vi "client_sw.vi"(5 "receive?":bool, 7 "data in":string, 8 "error constant":errorcluster, 11 "port":u16=6340) -> (0 "error constant 2":errorcluster, 3 "data out":string)   [LabVIEW 2015]
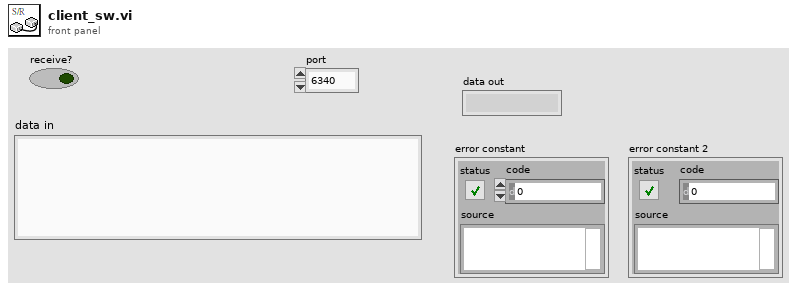
[diagram p1: front panel]
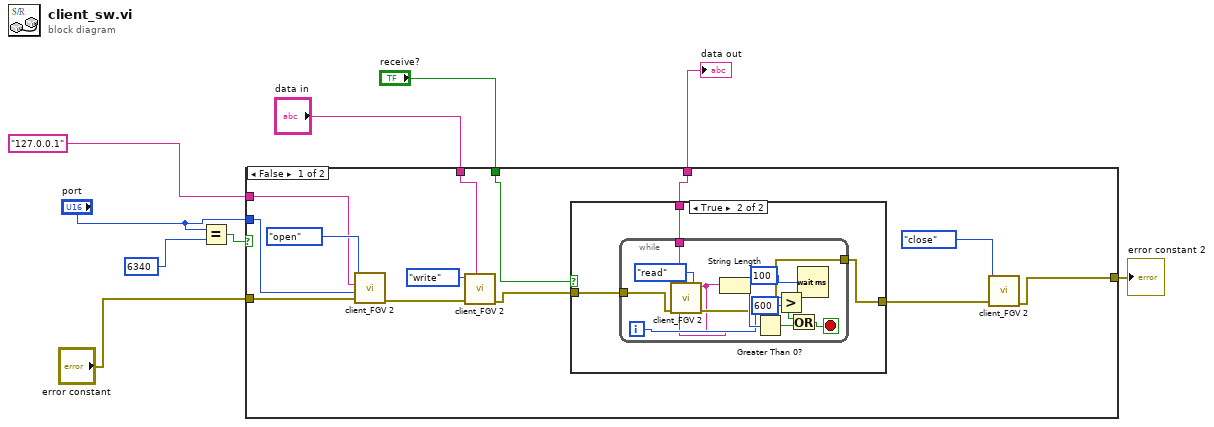
[diagram p0: block diagram]
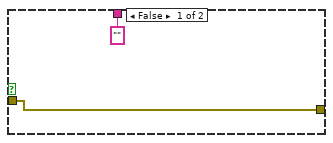
[diagram p2: hidden frame]
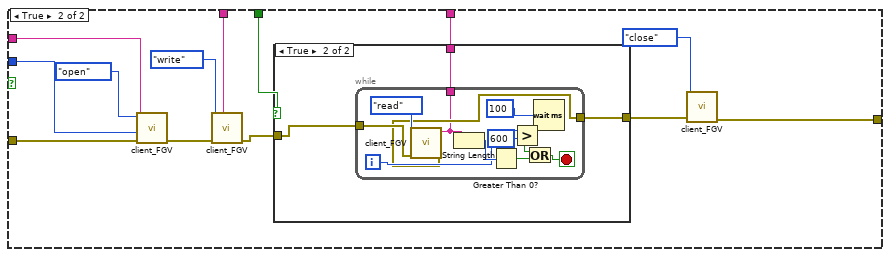
[diagram p3: hidden frame]
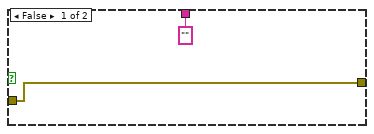
[diagram p4: hidden frame]
diagram:
  n1 = Equal?(x="port", y=u16 6340 ("port")) -> (x = y?=w8:bool)
  n2 = case shown="False" w8 {
    tunnel: "127.0.0.1" ("address") -> [w10 w51]
    tunnel: "port" -> [w11 w50]
    tunnel: "error constant" -> [w20 w49]
    tunnel: "data in" -> [w13 w46]
    tunnel: "receive?" -> [w14 w44]
    tunnel: [w12 w43] -> w2
    tunnel: [w15 w40] -> w1
    frame False {
      n3 = call "client_FGV 2.vi"("error constant"=w20, "port"=w11, "address"=w10, "Enum"=enum16{"open", "idle", "write", "read", "close"}."open") -> ("error constant 2"=w19:errorcluster)  [unwired: 6 in, 1 out]
      n4 = call "client_FGV 2.vi"("data in"=w13, "error constant"=w19, "Enum"=enum16{"open", "idle", "write", "read", "close"}."write") -> ("error constant 2"=w17:errorcluster)  [unwired: 7 in, 1 out]
      n5 = case shown="True" w14 {
        tunnel: w17 -> [w23 w27]
        tunnel: [w23 w26] -> w16
        tunnel: ["" ("data out") w25] -> w12
        frame False {
        }
        frame True {
          n6 = while {
            tunnel: w27 -> [w31]
            tunnel: [w29] -> w26
            tunnel: [w28] -> w25
            i -> [w33]
            stop <- w35 stop-if-true
            n7 = call "client_FGV 2.vi"("error constant"=w31, "Enum"=enum16{"open", "idle", "write", "read", "close"}."read") -> ("error constant 2"=w29:errorcluster, "data out"=w28:string)  [unwired: 8 in]
            n8 = String Length(string=w28) -> (length=w37:i32)
            n9 = Greater Than 0?(x=w37) -> (x > 0?=w36:bool)
            n10 = Greater?(x=w33, y=600) -> (0:w34:bool)
            n11 = Or(x=w34, y=w36) -> (x .or. y?=w35:bool)
            n12 = Wait (ms)(milliseconds to wait=u32 100) -> ()  [unwired: 1 out]
          }
        }
      }
      n13 = call "client_FGV 2.vi"("error constant"=w16, "Enum"=enum16{"open", "idle", "write", "read", "close"}."close") -> ("error constant 2"=w15:errorcluster)  [unwired: 8 in, 1 out]
    }
    frame True {
      n14 = call "client_FGV.vi"("error constant"=w49, "port"=w50, "address"=w51, "Enum"=enum16{"open", "idle", "write", "read", "close"}."open") -> ("error constant 2"=w48:errorcluster)  [unwired: 6 in, 1 out]
      n15 = call "client_FGV.vi"("data in"=w46, "error constant"=w48, "Enum"=enum16{"open", "idle", "write", "read", "close"}."write") -> ("error constant 2"=w45:errorcluster)  [unwired: 7 in, 1 out]
      n16 = case shown="True" w44 {
        tunnel: w45 -> [w53 w56]
        tunnel: ["" ("data out") w55] -> w43
        tunnel: [w53 w54] -> w42
        frame False {
        }
        frame True {
          n17 = while {
            tunnel: w56 -> [w67]
            tunnel: [w58] -> w54
            tunnel: [w57] -> w55
            i -> [w60]
            stop <- w62 stop-if-true
            n18 = call "client_FGV.vi"("error constant"=w67, "Enum"=enum16{"open", "idle", "write", "read", "close"}."read") -> ("error constant 2"=w58:errorcluster, "data out"=w57:string)  [unwired: 8 in]
            n19 = String Length(string=w57) -> (length=w64:i32)
            n20 = Greater Than 0?(x=w64) -> (x > 0?=w63:bool)
            n21 = Greater?(x=w60, y=600) -> (0:w61:bool)
            n22 = Or(x=w61, y=w63) -> (x .or. y?=w62:bool)
            n23 = Wait (ms)(milliseconds to wait=u32 100) -> ()  [unwired: 1 out]
          }
        }
      }
      n24 = call "client_FGV.vi"("error constant"=w42, "Enum"=enum16{"open", "idle", "write", "read", "close"}."close") -> ("error constant 2"=w40:errorcluster)  [unwired: 8 in, 1 out]
    }
  }
  "data out" <- w2
  "error constant 2" <- w1
